vi "Get tau_i, tau_phi, tau_m at Cursor.vi"(8 "Error In":errorcluster, 11 "Cursor Info":T1) -> (0 "Error Out":errorcluster, 1 "current tau_m":dbl[unit], 2 "current tau_ph":dbl[unit], 3 "tau_i":dbl[unit], 4 "original tau_ph":dbl[unit], 6 "original tau_m":dbl[unit])   [LabVIEW 2019]
uses:
  Cursor Info.ctl
  Phasor UC_N[W] Parameters.ctl
  SEPXP Phasor Plot Info.ctl
  Pseudo Phasor Parameters.ctl
  Phasor Explorer Display Parameters.ctl
  Type of Series.ctl
  Phasor Explorer Phasor Parameters.ctl
  Phasor Calculation Type.ctl
  Phasor Type.ctl
  Phasor Explorer Decay Parameters.ctl
  IRF Model.ctl
  Phasor Explorer Gate Parameters.ctl
  Gate Type.ctl
  Phasor Explorer Detector Parameters.ctl
  XY Graph Add-Ons.lvlib
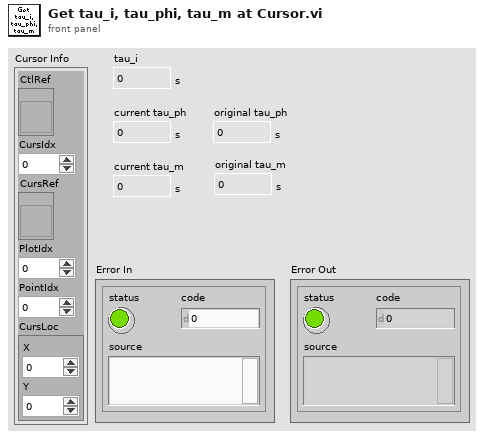
[diagram p1: front panel]
types:
  T1 = typedef "Cursor Info.ctl" = cluster{"CtlRef":refnum<vi>, "CursIdx":i32, "CursRef":refnum<vi>, "PlotIdx":i32, "PointIdx":i32, "CursLoc":cluster{"X":dbl, "Y":dbl}}
  T2 = typedef "Phasor UC_N[W] Parameters.ctl" = cluster{"Laser Period":dbl[unit], "Gate Width":dbl[unit], "Gate Step":dbl[unit], "Harmonic frequency":dbl[unit], "IRF offset":dbl[unit], "# Gates":dbl}
  T3 = typedef "Pseudo Phasor Parameters.ctl" = cluster{"Display Parameters":T4, "Phasor Parameters":T6, "Decay & IRF Parameters":T9, "Gate Parameters":T11, "Detector Parameters":T13}
  T4 = typedef "Phasor Explorer Display Parameters.ctl" = cluster{"# Points":i32, "Ramp Type":enum16{"Linear", "Logarithmic"}, "Type of Series":T5, "Min tau":dbl[unit], "Max tau":dbl[unit], "Include 0":bool, "Include Infinity":bool}
  T5 = typedef "Type of Series.ctl" = enum16{"1-Exp Decays", "Linear Combination of 1-Exp"}
  T6 = typedef "Phasor Explorer Phasor Parameters.ctl" = cluster{"Harmonic frequency":dbl[unit], "Use f* = 1/D Frequency":bool, "Calibrated Phasor":bool, "Calibration Lifetime":dbl[unit], "Phasor Calculation":T7, "SEPL Type":T8, "# Gates":dbl, "Square Gate Width":dbl[unit], "Show Ticks":bool}
  T7 = typedef "Phasor Calculation Type.ctl" = enum16{"Direct Sum", "Analytical Formula"}
  T8 = typedef "Phasor Type.ctl" = enum16{"UC", "L_N", "L_N[W]"}
  T9 = typedef "Phasor Explorer Decay Parameters.ctl" = cluster{"Lifetime":dbl[unit], "IRF Offset":dbl[unit], "Laser Period":dbl[unit], "Normalized Decays":bool, "IRF Model":T10, "IRF Parameter 1":dbl[unit]}
  T10 = typedef "IRF Model.ctl" = enum16{"Dirac", "Exponential"}
  T11 = typedef "Phasor Explorer Gate Parameters.ctl" = cluster{"First Gate Start":dbl[unit], "Use Gate Center":bool, "Gate Width":dbl[unit], "Gate Step":dbl[unit], "# Gates":dbl, "Gate Type":T12, "Edge Width":dbl[unit], "Top Slope":dbl[unit], "Reversed Sawtooth?":bool, "Analytical Computation":bool, "Tolerance":dbl, "Integration":enum32{"Item 0", "Item 1"}, "# Steps":dbl, "Type of User-defined Function":enum32{"Gate", "IRF"}}
  T12 = typedef "Gate Type.ctl" = enum16{"Square", "Finite Edge Square", "Finite Edge, Tilted Top Square", "Triangle", "Sawtooth", "User-defined"}
  T13 = typedef "Phasor Explorer Detector Parameters.ctl" = cluster{"Frames/Image":i32, "Gates/Frame":i32, "Bits/Frame":i32, "Multiplicity":i32, "Incident Signal":dbl}
  T14 = typedef "SEPXP Phasor Plot Info.ctl" = cluster{"Lifetime/Fraction Array":dbl[], "Phasor Explorer Parameters":T3, "Phase Lifetimes":dbl[], "Modulus Lifetimes":dbl[]}
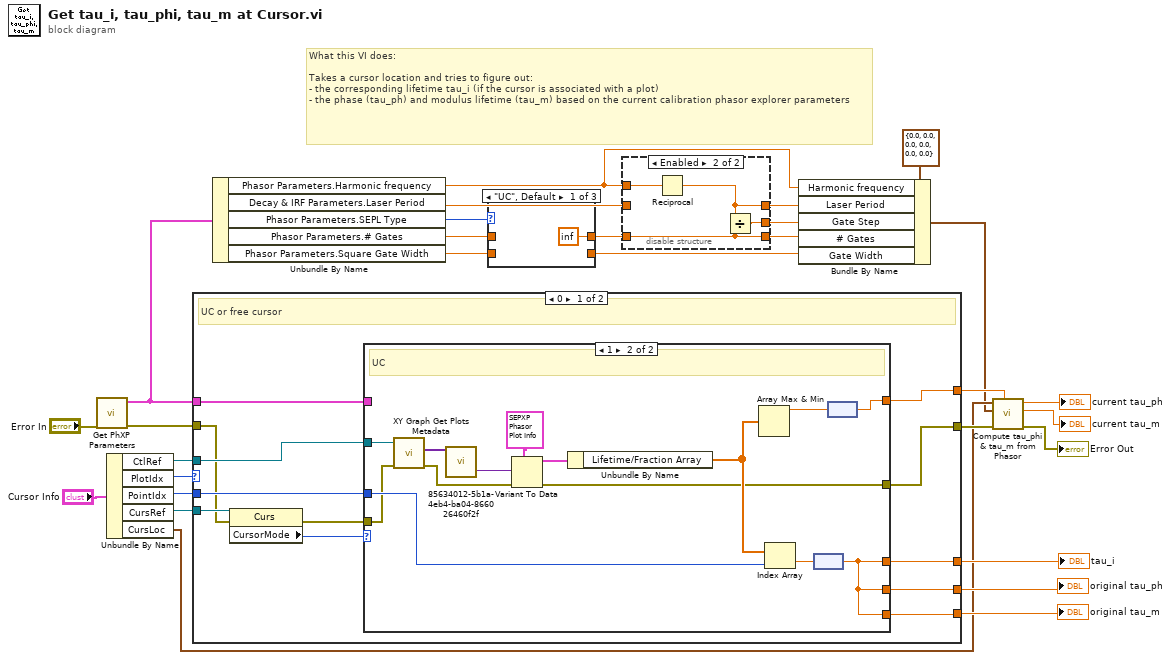
[diagram p0: block diagram]
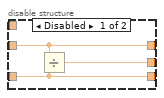
[diagram p2: hidden frame]
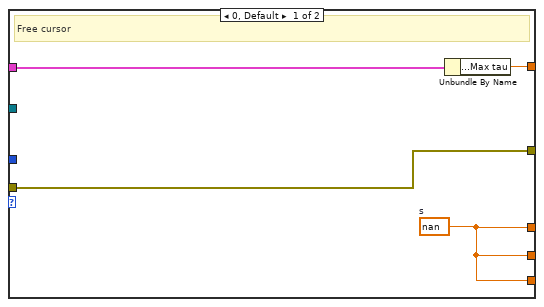
[diagram p5: hidden frame]
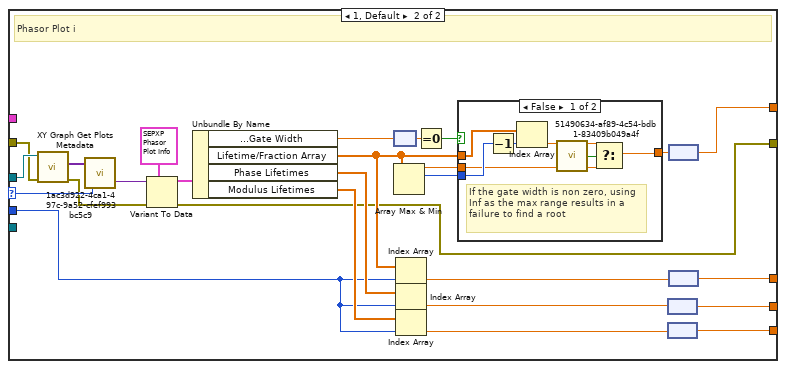
[diagram p6: hidden frame]
diagram:
  # "What this VI does:\n\nTakes a cursor location and tries to figure out:\n- the corresponding lifetime tau_i (if the cursor is associated with a plot)\n- the phase (tau_ph) and modulus lifetime (tau_m) based on the current calibration phasor explorer parameters"
  n1 = call "Get PhXP Parameters.vi"("Error In"="Error In") -> ("Error Out"=w16:errorcluster, "Phasor Explorer Parameters"=w14:T3)  [unwired: 7 in, 2 out]
  n2 = Unbundle By Name("Cursor Info") -> ("CtlRef"=w19:refnum<vi>, "PlotIdx"=w28:i32, "PointIdx"=w27:i32, "CursRef"=w20:refnum<vi>, "CursLoc"=w11:cluster{"X":dbl, "Y":dbl})
  n3 = case shown="0" w28 {
    selector: w28 -> [_ w72]
    tunnel: w27 -> [w41 w66]
    tunnel: [w40 w84] -> w26
    tunnel: [w36 w60] -> w23
    tunnel: [w35 w76] -> w2
    tunnel: w20 -> [w39 _]
    tunnel: w19 -> [w34 w73]
    tunnel: [w33 w63] -> w18
    tunnel: [w32 w62] -> w17
    tunnel: w16 -> [w30 w61]
    tunnel: w14 -> [w31 _]
    frame 0 {
      # "UC or free cursor"
      n4 = property class="Curs"(reference=w39, error in=w30) -> (error out=w37:errorcluster, "CursorMode"=w38:u32)  [unwired: 1 out]
      n5 = case shown="1" w38 {
        tunnel: w41 -> [_ w59]
        tunnel: [w44 w46] -> w40
        tunnel: w37 -> [w42 w47]
        tunnel: [w42 w48] -> w36
        tunnel: [w45 w55] -> w35
        tunnel: w34 -> [_ w54]
        tunnel: [w44 w46] -> w33
        tunnel: [w44 w46] -> w32
        tunnel: w31 -> [w43 _]
        frame 0, Default {
          w44 = dbl[unit] nan  # s
          # "Free cursor"
          n6 = Unbundle By Name(w43) -> ("Display Parameters.Max tau"=w45:dbl[unit])
        }
        frame 1 {
          # "UC"
          n7 = call "XY Graph Get Plots Metadata.vi"("Error In"=w47, "XYGraph Refnum"=w54) -> ("Error Out"=w49:errorcluster, "Plots Metadata"=w53:variant[])  [unwired: 6 in, 2 out]
          n8 = call "85634012-5b1a-4eb4-ba04-866026460f2f.vi"("1D Array"=w53) -> ("element"=w52:variant)  [unwired: 2 in]
          n9 = Variant To Data(error in=w49, type=T14 {"Lifetime/Fraction Array"=[], "Phasor Explorer Parameters"={"Display Parameters"={"# Points"=0, "Ramp Type"=enum."Linear", "Type of Series"=enum."1-Exp Decays", "Min tau"=0.0, "Max tau"=0.0, "Include 0"=FALSE, "Include Infinity"=FALSE}, "Phasor Parameters"={"Harmonic frequency"=0.0, "Use f* = 1/D Frequency"=FALSE, "Calibrated Phasor"=FALSE, "Calibration Lifetime"=1e-09, "Phasor Calculation"=enum."Direct Sum", "SEPL Type"=enum."UC", "# Gates"=1.0, "Square Gate Width"=1e-09, "Show Ticks"=FALSE}, "Decay & IRF Parameters"={"Lifetime"=0.0, "IRF Offset"=0.0, "Laser Period"=0.0, "Normalized Decays"=FALSE, "IRF Model"=enum."Dirac", "IRF Parameter 1"=0.0}, "Gate Parameters"={"First Gate Start"=0.0, "Use Gate Center"=FALSE, "Gate Width"=0.0, "Gate Step"=0.0, "# Gates"=0.0, "Gate Type"=enum."Square", "Edge Width"=0.0, "Top Slope"=0.0, "Reversed Sawtooth?"=FALSE, "Analytical Computation"=FALSE, "Tolerance"=1.0, "Integration"=enum."Item 0", "# Steps"=1.0, "Type of User-defined Function"=enum."Gate"}, "Detector Parameters"={"Frames/Image"=0, "Gates/Frame"=0, "Bits/Frame"=0, "Multiplicity"=0, "Incident Signal"=0.0}}, "Phase Lifetimes"=[], "Modulus Lifetimes"=[]} ("Phasor Graph Plot Info"), Variant=w52) -> (data=w50:T14, error out=w48:errorcluster)
          n10 = Unbundle By Name(w50) -> ("Lifetime/Fraction Array"=w57:dbl[])
          n11 = Array Max & Min(array=w57) -> (max value=w56:dbl)  [unwired: 3 out]
          n12 = Index Array(array=w57, index=w59) -> (element=w58:dbl)
          n13 = node(w58) -> (w46:dbl[unit])
          n14 = node(w56) -> (w55:dbl[unit])
        }
      }
    }
    frame 1, Default {
      # "Phasor Plot i"
      n15 = call "XY Graph Get Plots Metadata.vi"("Error In"=w61, "XYGraph Refnum"=w73) -> ("Error Out"=w69:errorcluster, "Plots Metadata"=w75:variant[])  [unwired: 6 in, 2 out]
      n16 = call "1ac3d922-4ca1-497c-9a52-cfef993bc5c9.vi"("index (0)"=w72, "1D Array"=w75) -> ("element"=w74:variant)  [unwired: 1 in]
      n17 = Variant To Data(error in=w69, type=T14 {"Lifetime/Fraction Array"=[], "Phasor Explorer Parameters"={"Display Parameters"={"# Points"=0, "Ramp Type"=enum."Linear", "Type of Series"=enum."1-Exp Decays", "Min tau"=0.0, "Max tau"=0.0, "Include 0"=FALSE, "Include Infinity"=FALSE}, "Phasor Parameters"={"Harmonic frequency"=0.0, "Use f* = 1/D Frequency"=FALSE, "Calibrated Phasor"=FALSE, "Calibration Lifetime"=1e-09, "Phasor Calculation"=enum."Direct Sum", "SEPL Type"=enum."UC", "# Gates"=1.0, "Square Gate Width"=1e-09, "Show Ticks"=FALSE}, "Decay & IRF Parameters"={"Lifetime"=0.0, "IRF Offset"=0.0, "Laser Period"=0.0, "Normalized Decays"=FALSE, "IRF Model"=enum."Dirac", "IRF Parameter 1"=0.0}, "Gate Parameters"={"First Gate Start"=0.0, "Use Gate Center"=FALSE, "Gate Width"=0.0, "Gate Step"=0.0, "# Gates"=0.0, "Gate Type"=enum."Square", "Edge Width"=0.0, "Top Slope"=0.0, "Reversed Sawtooth?"=FALSE, "Analytical Computation"=FALSE, "Tolerance"=1.0, "Integration"=enum."Item 0", "# Steps"=1.0, "Type of User-defined Function"=enum."Gate"}, "Detector Parameters"={"Frames/Image"=0, "Gates/Frame"=0, "Bits/Frame"=0, "Multiplicity"=0, "Incident Signal"=0.0}}, "Phase Lifetimes"=[], "Modulus Lifetimes"=[]} ("Phasor Graph Plot Info"), Variant=w74) -> (data=w70:T14, error out=w60:errorcluster)
      n18 = Unbundle By Name(w70) -> ("Phasor Explorer Parameters.Gate Parameters.Gate Width"=w83:dbl[unit], "Lifetime/Fraction Array"=w78:dbl[], "Phase Lifetimes"=w68:dbl[], "Modulus Lifetimes"=w67:dbl[])
      n19 = node(w83) -> (w82:dbl)
      n20 = Array Max & Min(array=w78) -> (max value=w80:dbl, max index (indices)=w79:i32)  [unwired: 2 out]
      n21 = Index Array(array=w78, index=w66) -> (element=w85:dbl)
      n22 = Index Array(array=w68, index=w66) -> (element=w65:dbl)
      n23 = Index Array(array=w67, index=w66) -> (element=w64:dbl)
      n24 = Equal To 0?(x=w82) -> (x = 0?=w81:bool)
      n25 = case shown="False" w81 {
        tunnel: w80 -> [w87 w93]
        tunnel: [w86 w93] -> w77
        tunnel: w79 -> [w90 _]
        tunnel: w78 -> [w91 _]
        frame False {
          # "If the gate width is non zero, using Inf as the max range results in a failure to find a root"
          n26 = Decrement(x=w90) -> (x-1=w89:i32)
          n27 = Index Array(array=w91, index=w89) -> (element=w88:dbl)
          n28 = call "51490634-af89-4c54-bdb1-83409b049a4f.vi"("Number"=w87) -> ("Is NaN or Inf?"=w92:bool)  [unwired: 8 in]
          n29 = Select(t=w88, s=w92, f=w87) -> (s? t:f=w86:dbl)
        }
        frame True {
        }
      }
      n30 = node(w65) -> (w63:dbl[unit])
      n31 = node(w64) -> (w62:dbl[unit])
      n32 = node(w77) -> (w76:dbl[unit])
      n33 = node(w85) -> (w84:dbl[unit])
    }
  }
  "tau_i" <- w26
  "original tau_ph" <- w18
  "original tau_m" <- w17
  n34 = Unbundle By Name(w14) -> ("Phasor Parameters.Harmonic frequency"=w6:dbl[unit], "Decay & IRF Parameters.Laser Period"=w13:dbl[unit], "Phasor Parameters.SEPL Type"=w10:T8, "Phasor Parameters.# Gates"=w9:dbl, "Phasor Parameters.Square Gate Width"=w4:dbl[unit])
  n35 = case shown="\"UC\", Default" w10 {
    tunnel: w9 -> [_ w95 w97]
    tunnel: [inf ("# Gates") w95 w97] -> w8
    tunnel: w4 -> [_ _ w96]
    tunnel: [_ _ w96] -> w3
    frame "UC", Default {
    }
    frame "L_N" {
    }
    frame "L_N[W]" {
    }
  }
  n36 = disable-structure shown="Enabled" {
    disable-tunnel: w13 -> [w99 _]
    disable-tunnel: [w100 w102] -> w12
    disable-tunnel: w8 -> [w98 w101]
    disable-tunnel: [w99 w103] -> w7
    disable-tunnel: w6 -> [_ w104]
    disable-tunnel: [w98 w101] -> w5
    frame Disabled {
      n37 = Divide(x=w99, y=w98) -> (x/y=w100:dbl[unit])
    }
    frame Enabled {
      n38 = Reciprocal(x=w104) -> (1/x=w103:dbl[unit])
      n39 = Divide(x=w103, y=w101) -> (x/y=w102:dbl[unit])
    }
  }
  n40 = Bundle By Name(cluster=T2 {"Laser Period"=0.0, "Gate Width"=0.0, "Gate Step"=0.0, "Harmonic frequency"=0.0, "IRF offset"=0.0, "# Gates"=0.0} ("Phasor UCN[W] Parameters"), "Harmonic frequency"=w6, "Laser Period"=w7, "Gate Step"=w12, "# Gates"=w5, "Gate Width"=w3) -> (w1:T2)
  n41 = call "Compute tau_phi & tau_m from Phasor.vi"("max tau"=w2, "Error In"=w23, "Phasor UCN[W] Parameters"=w1, "Phasor"=w11) -> ("Error Out"=→"Error Out":errorcluster, "tau_m"=→"current tau_m":dbl[unit], "tau_ph"=→"current tau_ph":dbl[unit])  [unwired: 5 in]
